vi "DSF.Transceiver.UDP.Tx.vi"(8 "error in (no error)":errorcluster, 9 "Transfer Tx parameters":T1, 10 "Transfer":refnum<class "DSF.Engine.Transfer.lvclass">, 11 "UDP Transceiver in":refnum<class "DSF.Transceiver.UDP.lvclass">) -> (0 "error out":errorcluster, 3 "UDP Transceiver out":refnum<class "DSF.Transceiver.UDP.lvclass">)   [LabVIEW 2017, in "DSF.Transceiver.UDP.lvlib" / "DSF.Transceiver.UDP.lvclass"]
uses:
  DSF.Transceiver.UDP.lvclass
  DSF.Transceiver.UDP.Parameters.Transfer.Tx.ctl
  Built/PharLap x86/Engine/c/DSF.Engine.lvlibp/Engine/Classes/Transfer/DSF.Engine.Transfer.lvclass
  DSF.Transceiver.UDP.lvclass/DSF.Transceiver.UDP.ctl
  Built/PharLap x86/Engine/c/DSF.Engine.lvlibp/Engine/Classes/Buffer/DSF.Engine.Memory.Buffer.Read.1D.U8.vi
  Built/PharLap x86/Engine/c/DSF.Engine.lvlibp/Engine/Classes/Buffer/DSF.Engine.Memory.Buffer.lvclass
  Built/PharLap x86/Dependencies/c/Memory Manager.lvlibp/1abvi3w/vi.lib/National Instruments/Memory Manager/Classes/Pointer/Memory.Pointer.lvclass
  C:/Git/DSF/DSF Core/Built/Windows/Engine/Memory Manager.lvlibp/1abvi3w/vi.lib/National Instruments/Memory Manager/Classes/Pointer/Memory.Pointer.lvclass
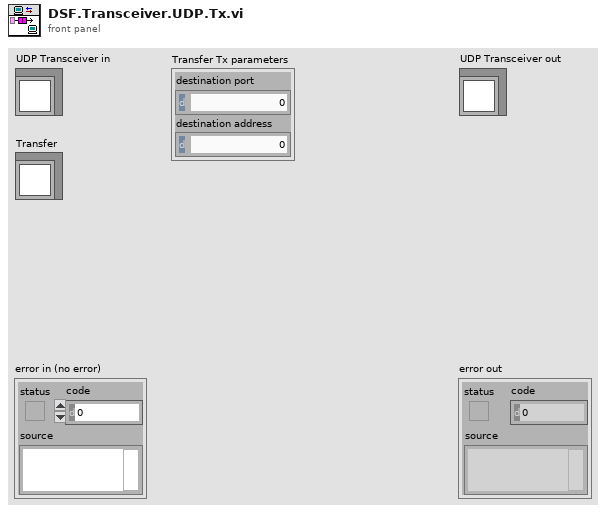
[diagram p1: front panel]
types:
  T1 = typedef "DSF.Transceiver.UDP.lvlib/DSF.Transceiver.UDP.lvclass/DSF.Transceiver.UDP.Parameters.Transfer.Tx.ctl" = cluster{"destination port":u16, "destination address":u32}
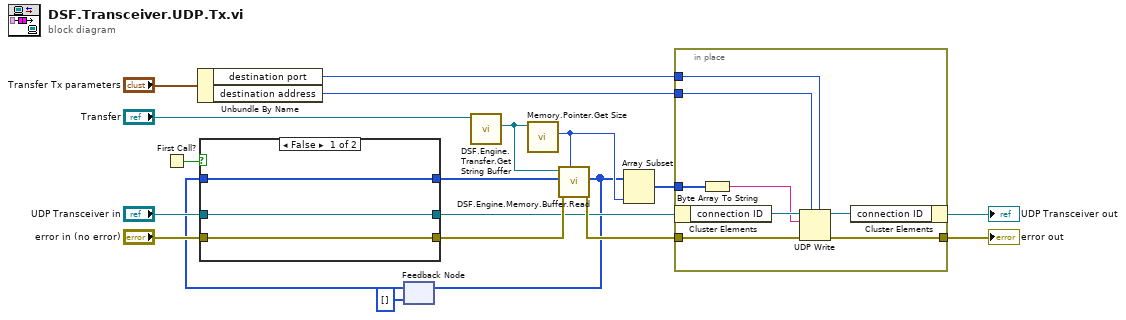
[diagram p0: block diagram]
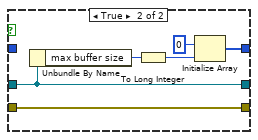
[diagram p2: hidden frame]
diagram:
  n1 = First Call?() -> (First Call?: T/F=w9:bool)
  n2 = Unbundle By Name("Transfer Tx parameters") -> ("destination port"=w15:u16, "destination address"=w16:u32)
  n3 = feedback #1(u8[] [] ("buffer out")) -> (w2:u8[])
  n4 = case shown="False" w9 {
    tunnel: "UDP Transceiver in" -> [w21 w27]
    tunnel: "error in (no error)" -> [w22 w28]
    tunnel: [w22 w28] -> w11
    tunnel: [w21 w27] -> w4
    tunnel: w2 -> [w20 _]
    tunnel: [w20 w24] -> w5
    frame False {
    }
    frame True {
      n5 = Unbundle By Name(w27) -> ("max buffer size"=w26:u64)
      n6 = To Long Integer(number=w26) -> (32bit integer=w23:i32)
      n7 = Initialize Array(u8 0 ("element"), w23) -> (w24:u8[])
    }
  }
  n8 = call "DSF.Engine.Transfer.Get String Buffer.vi"("Transfer in"="Transfer") -> ("Buffer"=w10:refnum<class "DSF.Engine.Memory.Buffer.lvclass">)  [unwired: 9 in, 1 out]
  n9 = call "Memory.Pointer.Get Size.vi"("Pointer in"=w10) -> ("size"=w8:u64)  [unwired: 9 in, 1 out]
  n10 = call-poly "DSF.Engine.Memory.Buffer.Read.vi"("count"=w8, "error in (no error)"=w11, "buffer in"=w5, "Buffer in"=w10) -> ("error out"=w13:errorcluster, "buffer out"=w1:u8[])  [unwired: 4 in, 2 out]
  n11 = feedback-in #1(w1) -> ()
  n12 = Array Subset(array=w1, length=w8) -> (w7:u8[])  [unwired: 1 in]
  n13 = in-place {
    in-place-border: w13 -> [w36]
    in-place-border: [w33] -> w19
    in-place-border: w16 -> [w32]
    in-place-border: w15 -> [w31]
    in-place-border: w7 -> [w30]
    n14 = in-place-cluster #2(w4) -> ("connection ID"=w35:refnum<k16>)
    n15 = Byte Array To String(unsigned byte array=w30) -> (string=w29:string)
    n16 = UDP Write(address=w32, port or service name=w31, connection ID=w35, data in=w29, 8:w36) -> (error out=w33:errorcluster, 3:w34:refnum<k16>)  [unwired: 1 in]
    n17 = in-place-cluster #2("connection ID"=w34) -> (→"UDP Transceiver out":refnum<class "DSF.Transceiver.UDP.lvclass">)
  }
  "error out" <- w19
